vi "Subsystem Logging.vi"   [LabVIEW 2016]
uses:
  Global Variables/Folder Names.vi
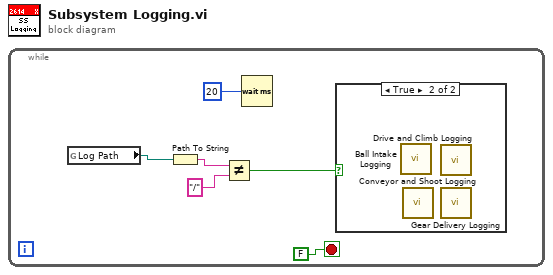
[diagram p0: block diagram]
diagram:
  n1 = while {
    stop <- FALSE stop-if-true
    n2 = global read "Folder Names.vi" "Log Path"() -> (w4:path)
    n3 = Path To String(path=w4) -> (string=w3:string)
    n4 = Not Equal?(x=w3, y="/") -> (x != y?=w1:bool)
    n5 = Wait (ms)(milliseconds to wait=20) -> ()  [unwired: 1 out]
    n6 = case shown="True" w1 {
      frame False {
      }
      frame True {
        n7 = call "Ball Intake Logging.vi"() -> ()  [unwired: 12 in]
        n8 = call "Conveyor and Shoot Logging.vi"() -> ()  [unwired: 12 in]
        n9 = call "Drive and Climb Logging.vi"() -> ()  [unwired: 12 in]
        n10 = call "Gear Delivery Logging.vi"() -> ()  [unwired: 12 in]
      }
    }
  }
